vi "키보드조종 쓰기부.vi"() -> ()   [LabVIEW 2014]
uses:
  <vilib>/Utility/inputDevices.llb/mouseAcquire.vi
  <vilib>/Utility/inputDevices.llb/closeMouse.vi
panel:
  out "숫자형 2":i32
  in  "정지":bool
  out "세로":i32
  out "가로":i32
  out "button info 4":T1 caption="버튼 정보"
  in  "key mode 4":enum16{"RELATIVE", "ABSOLUTE"}(ring)=enum."ABSOLUTE" caption="키 모드"
  out "문자 2":i16
  out "추가된 배열":i16[](array[numeric])
  out "문자열":string
  out "문자":i16=-19239
  out "플랫폼 조합키":T2
  out "조합키":cluster{"Num Pad":bool, "Menu Key":bool}
  out "Dato Leido":bool[](array[boolean])
  in  "stop 2":bool
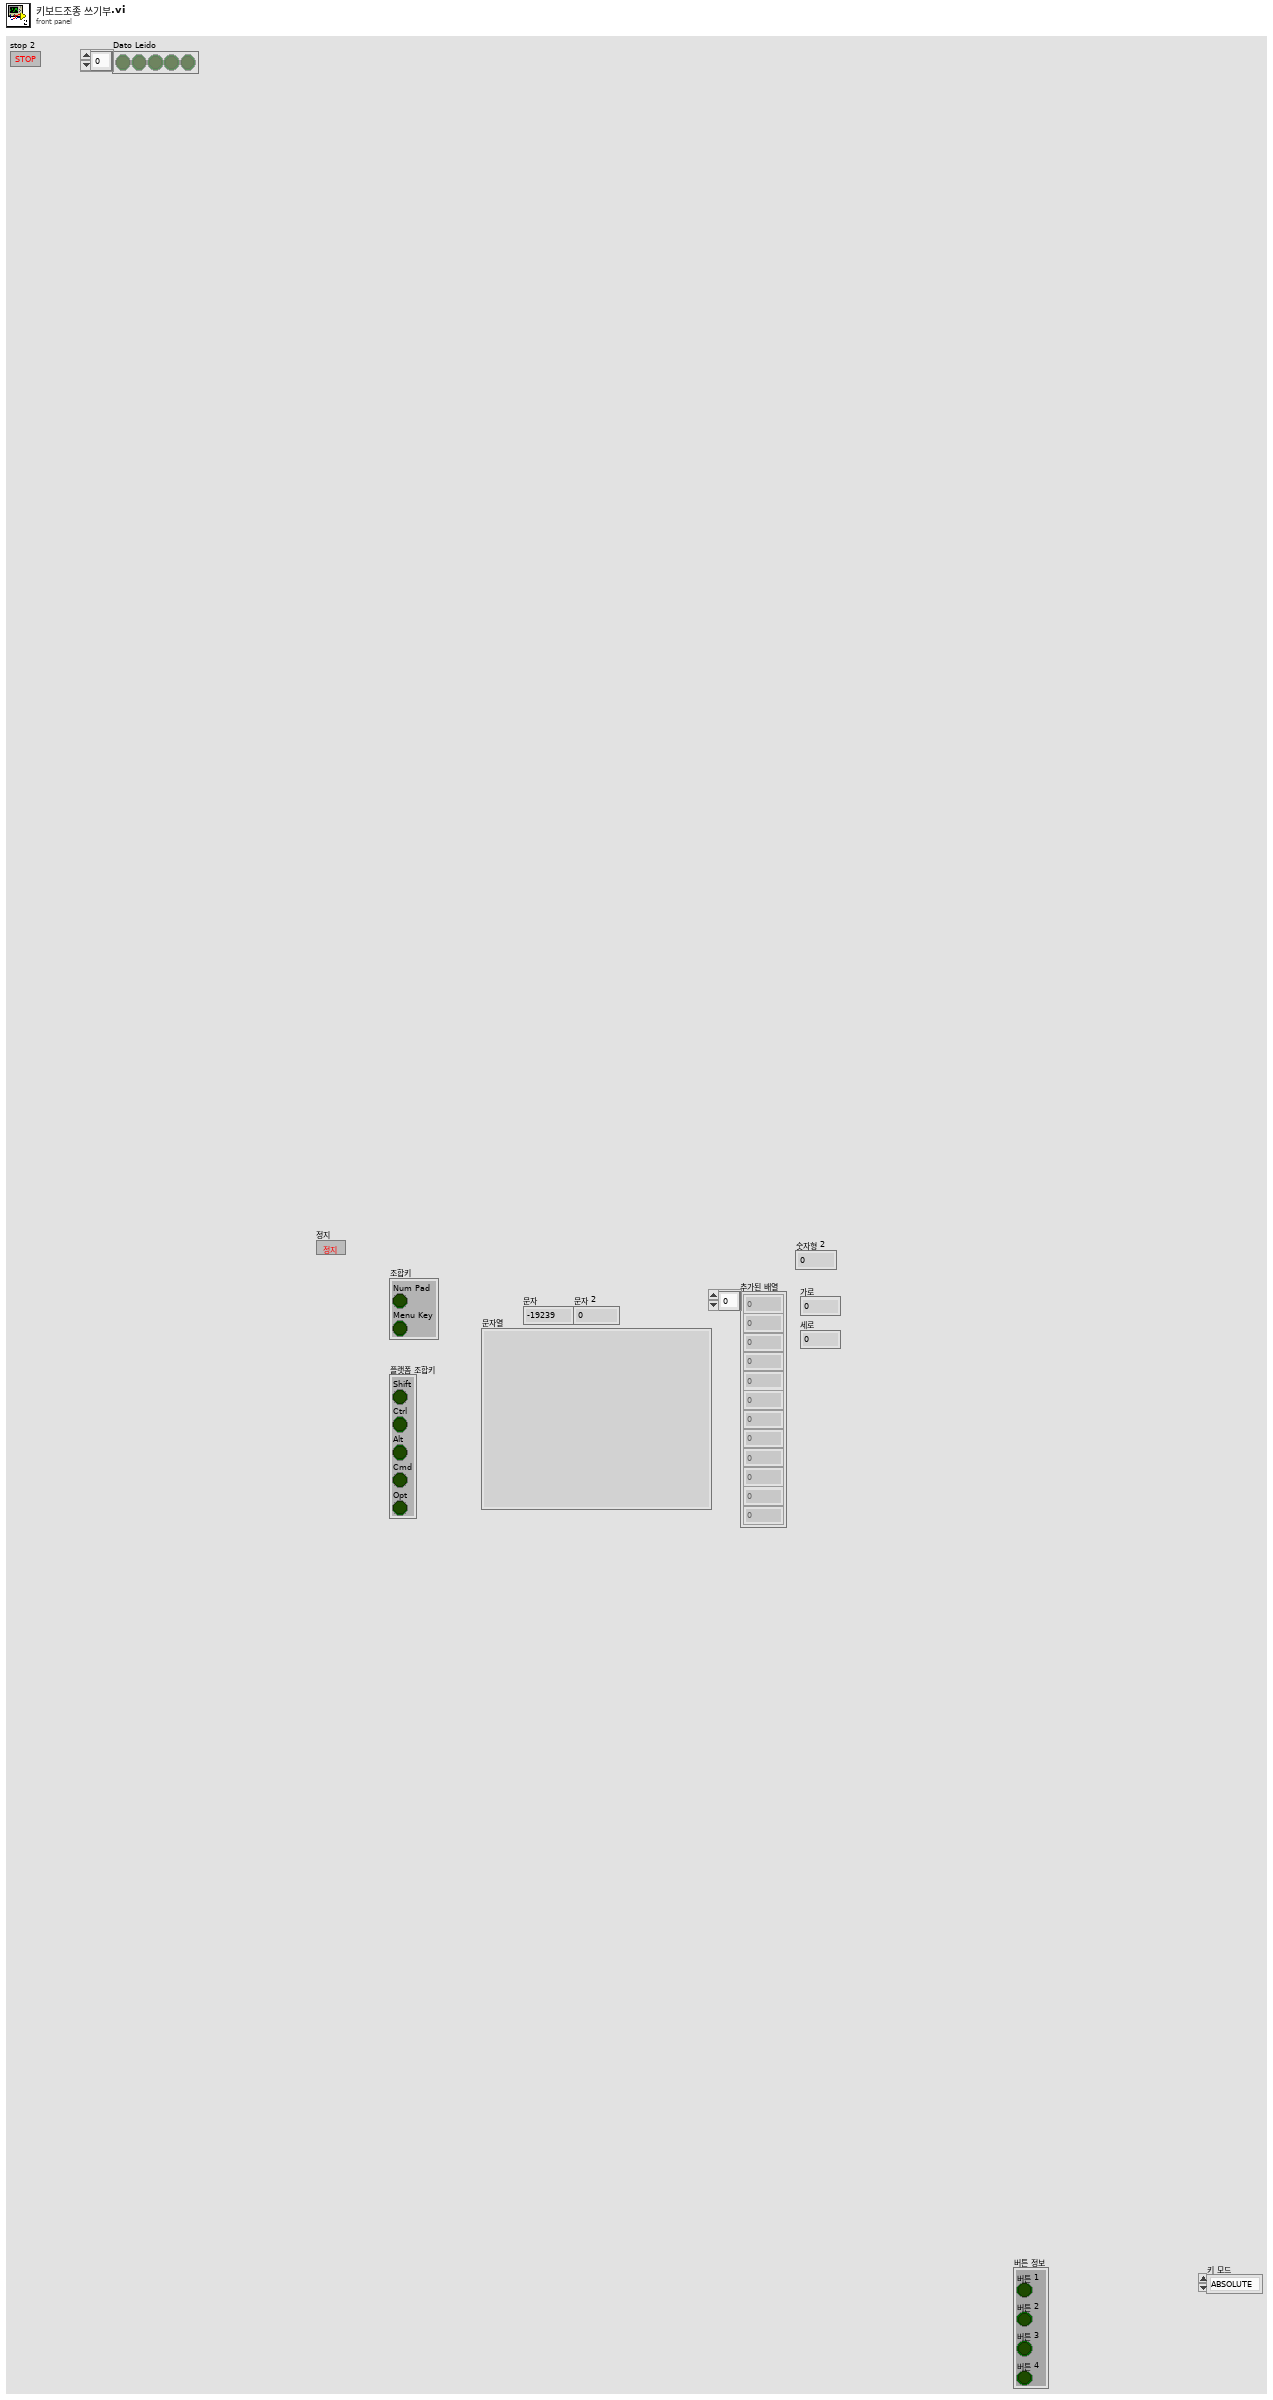
[diagram p1: front panel]
types:
  T1 = cluster{"button 1":bool, "button 2":bool, "button 3":bool, "button 4":bool}
  T2 = cluster{"Shift":bool, "Ctrl":bool, "Alt":bool, "Cmd":bool, "Opt":bool}
  T3 = cluster{"Horizontal":i32, "Vertical":i32, "Scrolling":i32}
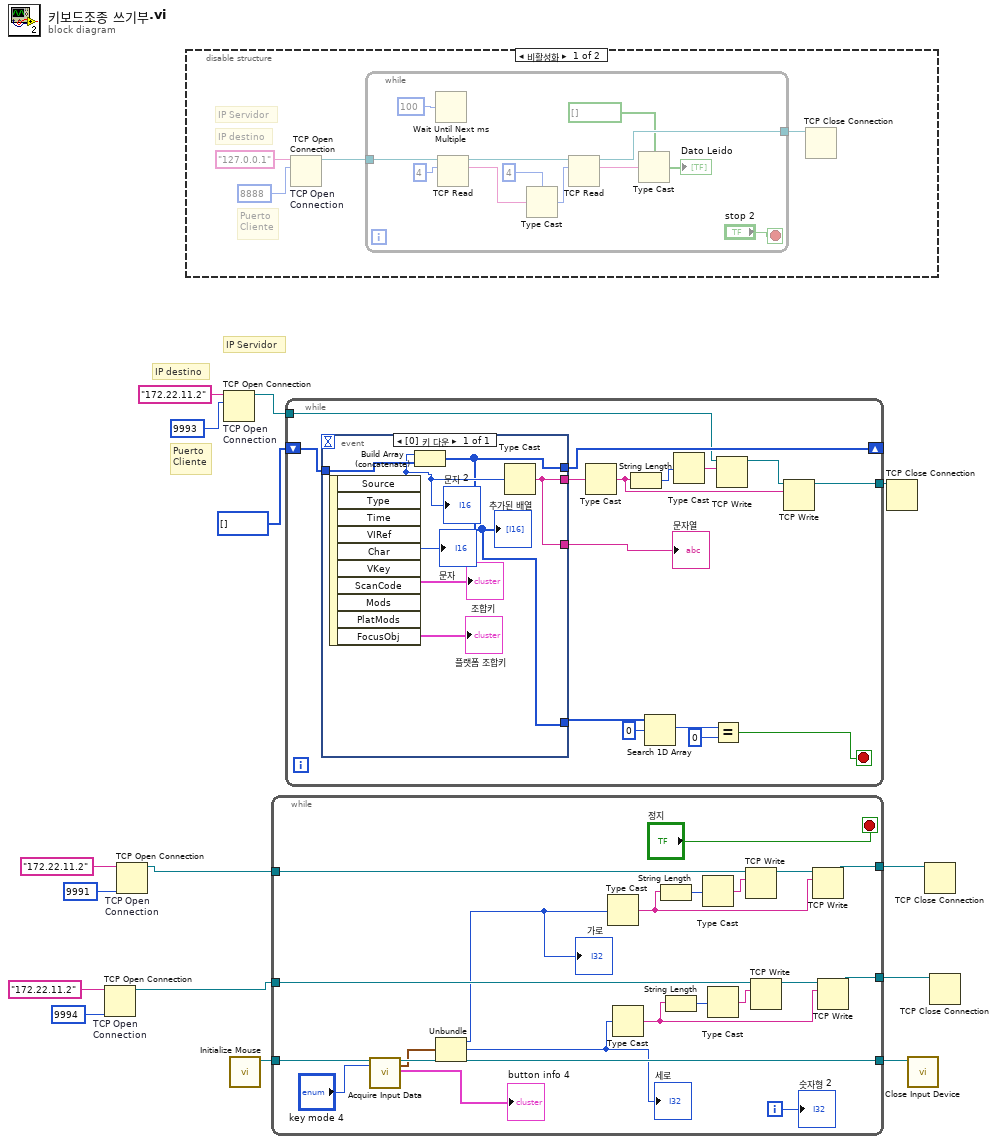
[diagram p0: block diagram]
diagram:
  # "Puerto\nCliente"
  # "IP Servidor"
  # "IP destino"
  n1 = TCP Open Connection "TCP Open \nConnection"(address="172.22.11.2" ("주소"), remote port or service name=u16 9994 ("원격 포트 또는 서비스 이름")) -> (connection ID=w1:refnum<k5>)  [unwired: 3 in, 1 out]
  n2 = TCP Open Connection "TCP Open \nConnection"(address="172.22.11.2" ("주소"), remote port or service name=u16 9991 ("원격 포트 또는 서비스 이름")) -> (connection ID=w2:refnum<k5>)  [unwired: 3 in, 1 out]
  n3 = disable-structure shown="비활성화" {
    frame Disabled {
      # "Puerto\nCliente"
      # "IP Servidor"
      # "IP destino"
      n4 = TCP Open Connection "TCP Open \nConnection"(address="127.0.0.1", remote port or service name=u16 8888) -> (connection ID=w16:refnum<k5>)  [unwired: 3 in, 1 out]
      n5 = while {
        tunnel: w16 -> [w31]
        tunnel: [w29] -> w17
        stop <- "stop 2" stop-if-true
        n6 = Wait Until Next ms Multiple(millisecond multiple=u32 100) -> ()  [unwired: 1 out]
        n7 = TCP Read(connection ID=w31, bytes to read=4) -> (connection ID out=w30:refnum<k5>, data out=w26:string)  [unwired: 3 in, 1 out]
        n8 = Type Cast(type=4 ("bytes to read"), x=w26) -> (*(type *) &x=w25:i32)
        n9 = TCP Read(connection ID=w30, bytes to read=w25) -> (connection ID out=w29:refnum<k5>, data out=w24:string)  [unwired: 3 in, 1 out]
        n10 = Type Cast(type=bool[] [] ("Dato array"), x=w24) -> (*(type *) &x=→"Dato Leido":bool[])
      }
      n11 = TCP Close Connection(connection ID=w17) -> ()  [unwired: 2 in, 2 out]
    }
    frame Enabled {
    }
  }
  n12 = TCP Open Connection "TCP Open \nConnection"(address="172.22.11.2", remote port or service name=u16 9993) -> (connection ID=w7:refnum<k5>)  [unwired: 3 in, 1 out]
  n13 = call <vilib>:"Initialize Mouse.vi"() -> ("device ID"=w12:refnum<k1>)  [unwired: 10 in, 1 out]
  n14 = while {
    tunnel: [w46] -> w13
    tunnel: w12 -> [w45]
    tunnel: w2 -> [w44]
    tunnel: [w43] -> w11
    tunnel: w1 -> [w40]
    tunnel: [w41] -> w10
    i -> [w32]
    stop <- "정지" stop-if-true
    n15 = call-poly <vilib>:"Acquire Input Data.vi"("device ID"=w45, "key mode"="key mode 4") -> ("device ID"=w46:refnum<k1>, "axis info"=w42:T3, "button info"=→"button info 4":T1)  [unwired: 14 in, 1 out]
    n16 = Unbundle(w42) -> ("Horizontal"=w35:i32, "Vertical"=w34:i32)  [unwired: 1 out]
    "가로" <- w35
    "세로" <- w34
    n17 = Type Cast(x=w35) -> (*(type *) &x=w50:string)  [unwired: 1 in]
    n18 = Type Cast(x=w34) -> (*(type *) &x=w36:string)  [unwired: 1 in]
    n19 = String Length(string=w50) -> (length=w49:i32)
    n20 = String Length(string=w36) -> (length=w37:i32)
    n21 = Type Cast(x=w49) -> (*(type *) &x=w48:string)  [unwired: 1 in]
    n22 = Type Cast(x=w37) -> (*(type *) &x=w38:string)  [unwired: 1 in]
    n23 = TCP Write(connection ID=w44, data in=w48) -> (connection ID out=w47:refnum<k5>)  [unwired: 2 in, 2 out]
    n24 = TCP Write(connection ID=w40, data in=w38) -> (connection ID out=w39:refnum<k5>)  [unwired: 2 in, 2 out]
    n25 = TCP Write(connection ID=w47, data in=w50) -> (connection ID out=w43:refnum<k5>)  [unwired: 2 in, 2 out]
    n26 = TCP Write(connection ID=w39, data in=w36) -> (connection ID out=w41:refnum<k5>)  [unwired: 2 in, 2 out]
    "숫자형 2" <- w32
  }
  n27 = while {
    tunnel: w7 -> [w58]
    tunnel: [w63] -> w14
    shift-right: [w61] -> _
    shift-left: i16[] [] -> [w62]
    stop <- w53 stop-if-true
    n28 = event shown="[0] 키 다운" {
      selector: _ -> [_]
      dyn-events: _ -> [_]
      timeout: _ -> [_]
      tunnel: [w68] -> w61
      tunnel: w62 -> [w71]
      tunnel: [w70] -> w60
      tunnel: [w70] -> w59
      tunnel: [w68] -> w57
      event Key Down {
        n29 = event-data() -> ("Char"=w69:i16, "Mods"=→"조합키":cluster{"Num Pad":bool, "Menu Key":bool}, "PlatMods"=→"플랫폼 조합키":T2)  [unwired: 1 in, 7 out]
        "문자" <- w69
        "문자 2" <- w69
        n30 = Build Array (concatenate)(w69, w71) -> (w68:i16[])
        "추가된 배열" <- w68
        n31 = Type Cast(x=w69) -> (*(type *) &x=w70:string)  [unwired: 1 in]
      }
    }
    "문자열" <- w60
    n32 = Type Cast(x=w59) -> (*(type *) &x=w64:string)  [unwired: 1 in]
    n33 = String Length(string=w64) -> (length=w65:i32)
    n34 = Search 1D Array(1D array=w57, element=i16 0 ("원소")) -> (index of element=w55:i32)  [unwired: 1 in]
    n35 = Type Cast(x=w65) -> (*(type *) &x=w66:string)  [unwired: 1 in]
    n36 = Equal?(x=w55, y=0) -> (x = y?=w53:bool)
    n37 = TCP Write(connection ID=w58, data in=w66) -> (connection ID out=w67:refnum<k5>)  [unwired: 2 in, 2 out]
    n38 = TCP Write(connection ID=w67, data in=w64) -> (connection ID out=w63:refnum<k5>)  [unwired: 2 in, 2 out]
  }
  n39 = TCP Close Connection(connection ID=w14) -> ()  [unwired: 2 in, 2 out]
  n40 = call-poly <vilib>:"Close Input Device.vi"("device ID"=w13) -> ()  [unwired: 9 in, 1 out]
  n41 = TCP Close Connection(connection ID=w11) -> ()  [unwired: 2 in, 2 out]
  n42 = TCP Close Connection(connection ID=w10) -> ()  [unwired: 2 in, 2 out]
